vi "client.vi"() -> ()   [LabVIEW 2020]
panel:
  in  "设备信息":T1
  in  "停止":bool
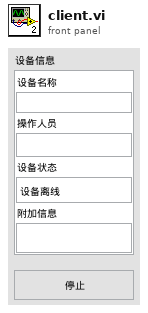
[diagram p1: front panel]
types:
  T1 = cluster{"设备名称":string, "操作人员":string, "设备状态":enum16{"设备离线", "设备正常", "设备缺料", "设备故障", "质量报警"}, "附加信息":string}
  T2 = cluster{"设备名称":bool, "操作人员":bool, "设备状态":bool, "附加信息":bool}
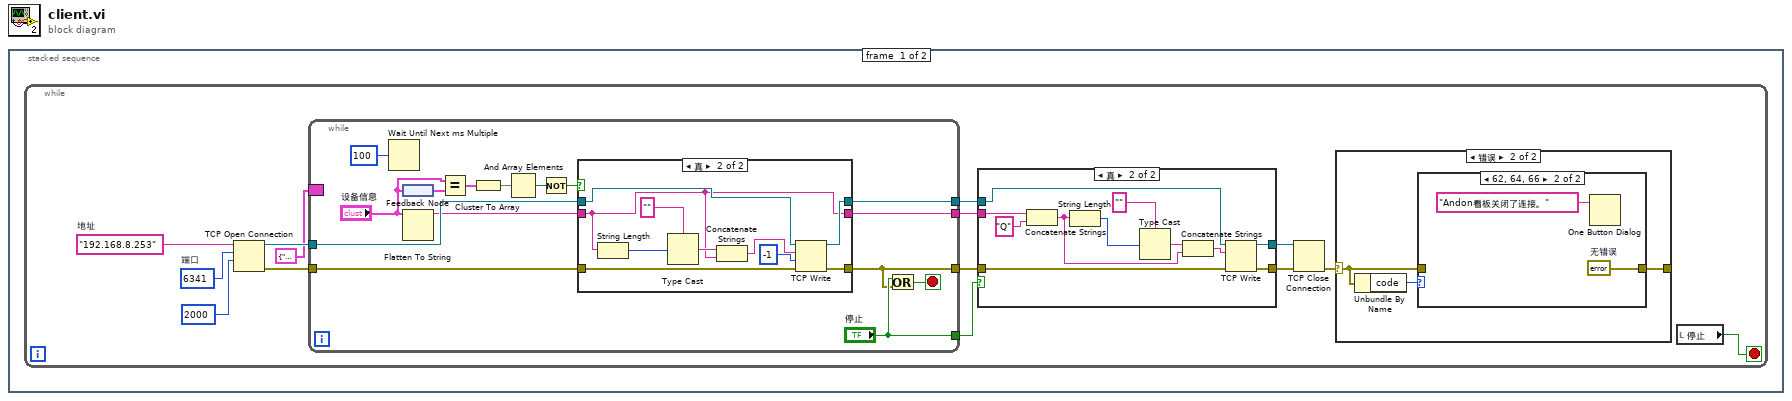
[diagram p0: block diagram]
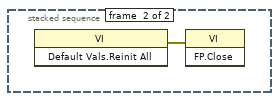
[diagram p6: hidden frame]
diagram:
  n1 = stacked-sequence {
    frame #0 {
      n2 = while {
        stop <- w1 stop-if-true
        w3 = u16 6341  # 端口
        w4 = "192.168.8.253"  # 地址
        n3 = TCP Open Connection(address=w4, remote port or service name=w3, timeout ms (60000)=2000 ("超时毫秒(60000)")) -> (connection ID=w14:refnum<k5>, error out=w13:errorcluster)  [unwired: 1 in, 1 out]
        n4 = while {
          tunnel: ["停止"] -> w8
          tunnel: [w34] -> w12
          tunnel: [w31] -> w10
          tunnel: w13 -> [w35]
          tunnel: w14 -> [w36]
          tunnel: [w24] -> w6
          border: T1 {"设备名称"="", "操作人员"="", "设备状态"=enum."设备正常", "附加信息"=""} ("设备信息") -> [_]
          stop <- w33 stop-if-true
          n5 = Wait Until Next ms Multiple(millisecond multiple=u32 100 ("毫秒倍数")) -> ()  [unwired: 1 out]
          n6 = feedback-in #1("设备信息") -> ()
          n7 = feedback #1() -> (w28:T1)
          n8 = Flatten To String(anything="设备信息") -> (data string=w25:string)  [unwired: 3 in, 2 out]
          n9 = Equal?(x="设备信息", y=w28) -> (x = y?=w27:T2)
          n10 = Cluster To Array(cluster=w27) -> (array=w26:bool[])
          n11 = And Array Elements(Boolean array=w26) -> (logical AND=w23:bool)
          n12 = Not(x=w23) -> (.not. x?=w22:bool)
          n13 = case shown="真" w22 {
            tunnel: w36 -> [w39 w49]
            tunnel: w35 -> [w38 w48]
            tunnel: [w39 w47] -> w34
            tunnel: [w38 w46] -> w31
            tunnel: w25 -> [w37 w40]
            tunnel: [w37 w40] -> w24
            frame False {
            }
            frame True {
              n14 = String Length(string=w40) -> (length=w44:i32)
              n15 = Type Cast(type="", x=w44) -> (*(type *) &x=w42:string)
              n16 = Concatenate Strings(w42, w40) -> (w41:string)
              n17 = TCP Write(connection ID=w49, data in=w41, error in (no error)=w48, 9:-1) -> (connection ID out=w47:refnum<k5>, error out=w46:errorcluster)  [unwired: 1 out]
            }
          }
          n18 = Or(x="停止", y=w31) -> (x .or. y?=w33:bool)
        }
        n19 = case shown="真" w8 {
          tunnel: w12 -> [w51 w62]
          tunnel: [w51 w60] -> w11
          tunnel: w10 -> [w50 w61]
          tunnel: [w50 w59] -> w9
          tunnel: w6 -> [_ w57]
          frame False {
          }
          frame True {
            n20 = Concatenate Strings(w57, "Q") -> (w53:string)
            n21 = String Length(string=w53) -> (length=w56:i32)
            n22 = Type Cast(type="", x=w56) -> (*(type *) &x=w54:string)
            n23 = Concatenate Strings(w54, w53) -> (w52:string)
            n24 = TCP Write(connection ID=w62, data in=w52, error in (no error)=w61) -> (connection ID out=w60:refnum<k5>, error out=w59:errorcluster)  [unwired: 2 out]
          }
        }
        n25 = TCP Close Connection(connection ID=w11, error in (no error)=w9) -> (error out=w7:errorcluster)  [unwired: 2 out]
        n26 = case shown="错误" w7 {
          selector: w7 -> [w15 w17]
          tunnel: [w15 w16] -> _
          frame No Error {
          }
          frame Error {
            n27 = Unbundle By Name(w17) -> ("code"=w18:i32)
            n28 = case shown="62, 64, 66" w18 {
              tunnel: w17 -> [w19 _]
              tunnel: [w19 w21] -> w16
              frame Default {
              }
              frame 62, 64, 66 {
                w21 = errorcluster {"status"=FALSE, "code"=0, "source"=""}  # 无错误
                n29 = One Button Dialog(message="Andon看板关闭了连接。" ("服务器关闭")) -> ()  [unwired: 1 in, 1 out]
              }
            }
          }
        }
        n30 = local read "停止"() -> (w1:bool)
      }
    }
    frame #1 {
      n31 = invoke class="VI" method="Default Vals.Reinit All"() -> (error out=w63:errorcluster)  [unwired: 3 in, 2 out]
      n32 = invoke class="VI" method="FP.Close"(error in=w63) -> ()  [unwired: 2 in, 3 out]
    }
  }
